vi "AutoAddEdge.vi"(0 "FSM in":refnum<class "FSM.Graph.lvclass">, 5 "sourceIndex":i32, 7 "targetIndex":i32, 9 "edgeSpec":string, 11 "error in (no error)":errorcluster, 12 "Point":cluster{"X":i16, "Y":i16}) -> (4 "FSM out":refnum<class "FSM.Graph.lvclass">, 6 "edgeIndex":i32, 15 "error out":errorcluster)   [LabVIEW 2015, in "FSM.Graph.lvclass"]
uses:
  FSM.Graph.lvclass
  FSM.Graph.lvclass/FSM.Graph.ctl
  FSM.Node/FSM.Node.lvclass
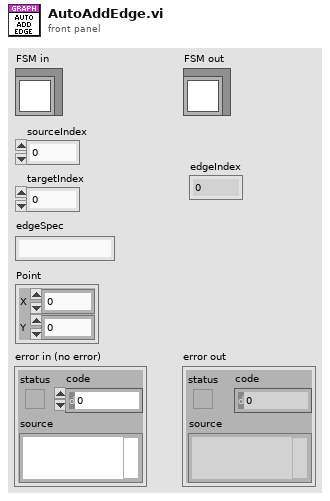
[diagram p1: front panel]
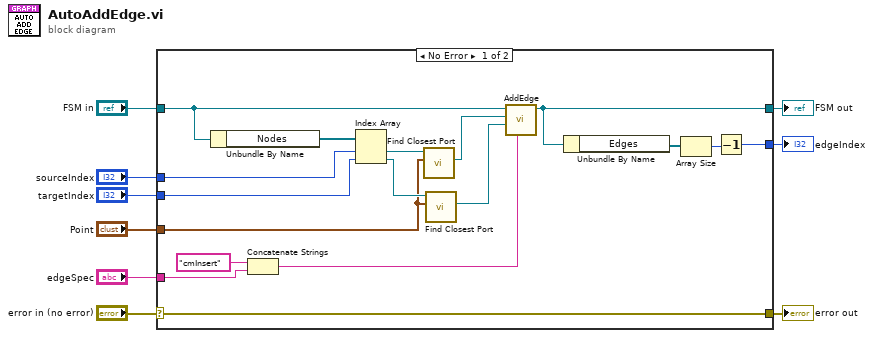
[diagram p0: block diagram]
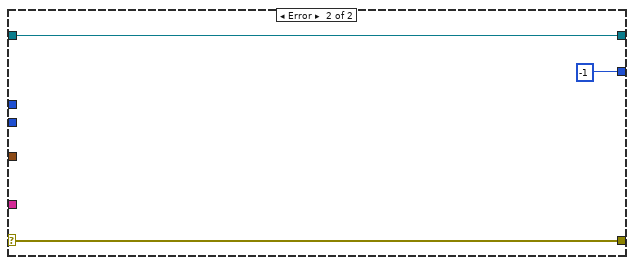
[diagram p2: hidden frame]
diagram:
  n1 = case shown="No Error" "error in (no error)" {
    selector: "error in (no error)" -> [w26 w29]
    tunnel: [w26 w29] -> w8
    tunnel: [w12 w28] -> w6
    tunnel: "FSM in" -> [w22 w28]
    tunnel: "edgeSpec" -> [w25 _]
    tunnel: "sourceIndex" -> [w20 _]
    tunnel: "targetIndex" -> [w19 _]
    tunnel: "Point" -> [w11 _]
    tunnel: [w10 -1] -> w1
    frame No Error {
      n2 = Unbundle By Name(w22) -> ("Nodes"=w21:refnum<class "FSM.Node.lvclass">[])
      n3 = Concatenate Strings("cmInsert" ("string"), w25) -> (w23:string)
      n4 = Index Array(array=w21, index #1=w20, index #2=w19) -> (element #1=w18:refnum<class "FSM.Node.lvclass">, element #2=w17:refnum<class "FSM.Node.lvclass">)
      n5 = call "Find Closest Port.vi"("point"=w11, "FSM.Node in"=w18) -> ("Port"=w16:refnum<class "FSM.Port.lvclass">)  [unwired: 6 in, 3 out]
      n6 = call "Find Closest Port.vi"("point"=w11, "FSM.Node in"=w17) -> ("Port"=w15:refnum<class "FSM.Port.lvclass">)  [unwired: 6 in, 3 out]
      n7 = call "AddEdge.vi"("edgeSpec"=w23, "Target Port"=w15, "Source Port"=w16, "FSM in"=w22) -> ("FSM out"=w12:refnum<class "FSM.Graph.lvclass">)  [unwired: 5 in, 2 out]
      n8 = Unbundle By Name(w12) -> ("Edges"=w14:refnum<class "FSM.Edge.lvclass">[])
      n9 = Array Size(array=w14) -> (size(s)=w13:i32)
      n10 = Decrement(x=w13) -> (x-1=w10:i32)
    }
    frame Error {
    }
  }
  "error out" <- w8
  "FSM out" <- w6
  "edgeIndex" <- w1
